vi "Configure.vi"(8 "error in (no error)":errorcluster, 11 "DemoStage in":refnum<class "DemoStage.lvclass">) -> (0 "error out":errorcluster, 3 "DemoStage out":refnum<class "DemoStage.lvclass">)   [LabVIEW 2020, in "DemoStage.lvlib" / "DemoStage.lvclass"]
uses:
  DemoStage.lvclass
  DemoStage.lvclass/DemoStage.ctl
  Hardware Abstraction Layer/Component/Stage/Stage/Stage.lvclass
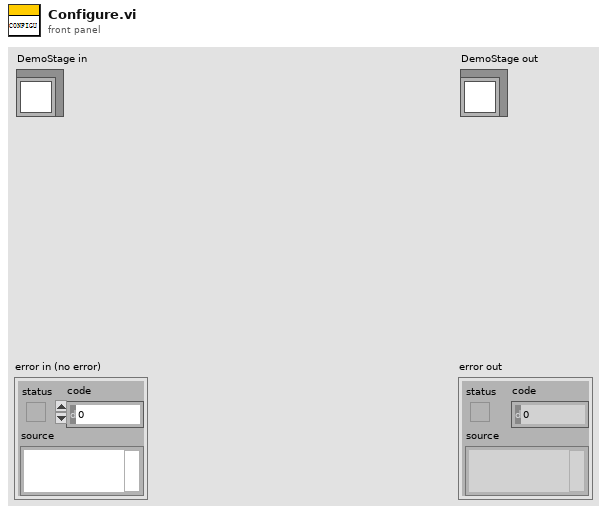
[diagram p1: front panel]
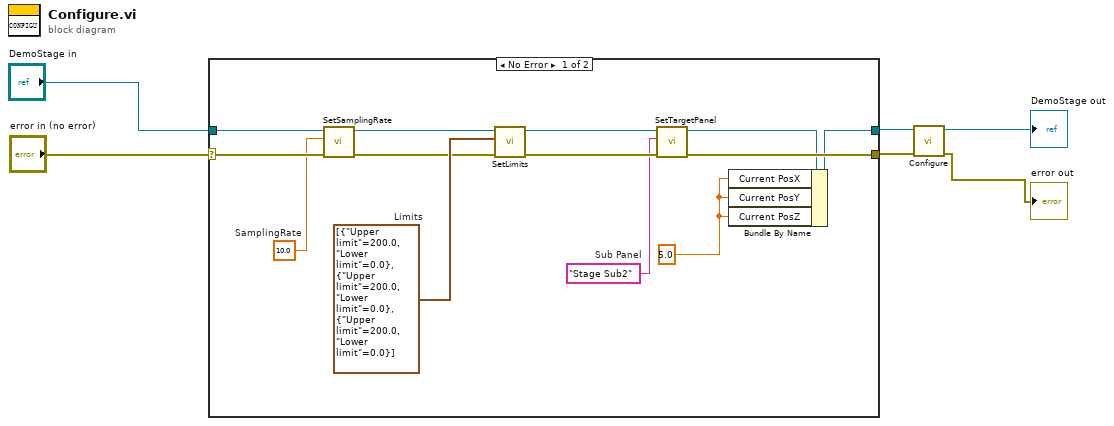
[diagram p0: block diagram]
diagram:
  n1 = case shown="No Error" "error in (no error)" {
    selector: "error in (no error)" -> [w19 w21]
    tunnel: [w14 w21] -> w3
    tunnel: [w8 w20] -> w4
    tunnel: "DemoStage in" -> [w9 w20]
    frame No Error {
      w7 = 5.0 ("Current PosZ")
      w10 = 10.0  # SamplingRate
      w15 = "Stage Sub2"  # Sub Panel
      w18 = cluster{"Upper limit":dbl, "Lower limit":dbl}[] [{"Upper limit"=200.0, "Lower limit"=0.0}, {"Upper limit"=200.0, "Lower limit"=0.0}, {"Upper limit"=200.0, "Lower limit"=0.0}]  # Limits
      n2 = call-dynamic "SetSamplingRate.vi"("error in (no error)"=w19, "SamplingRate(Hz)"=w10, "Device in"=w9) -> ("error out"=w12:errorcluster, "Device out"=w11:refnum<class "DemoStage.lvclass">)  [unwired: 7 in]
      n3 = call-dynamic "SetLimits.vi"("error in (no error)"=w12, "Limits"=w18, "Stage in"=w11) -> ("error out"=w17:errorcluster, "Stage out"=w16:refnum<class "DemoStage.lvclass">)  [unwired: 7 in]
      n4 = call-dynamic "SetTargetPanel.vi"("error in (no error)"=w17, "TargetPanel"=w15, "GRMActor in"=w16) -> ("error out"=w14:errorcluster, "GRMActor out"=w13:refnum<class "DemoStage.lvclass">)  [unwired: 7 in]
      n5 = Bundle By Name(cluster=w13, "Current PosX"=w7, "Current PosY"=w7, "Current PosZ"=w7) -> (w8:refnum<class "DemoStage.lvclass">)
    }
    frame Error {
    }
  }
  n6 = call-parent "Configure.vi"("error in (no error)"=w3, "Device in"=w4) -> ("error out"=→"error out":errorcluster, "Device out"=→"DemoStage out":refnum<class "DemoStage.lvclass">)  [unwired: 8 in]
